vi "Update Overlay.vi"(0 "CaliperType_w_Pic":T9 items=["Distance", "Mid Point", "Perpendicular Projection", "Lines Intersection", "Angle from Horizontal", "Angle from Vertical", "Angle Defined by 3 Points", "Angle Defined by 4 Points", "Bissecting Line", "Mid Line", "Center of Mass", "Area", "Line Fit", "Circle Fit", "Ellipse Fit"], 1 "Vision_Image 2":T2(plugin-control), 5 "Analysis_Point_Result Out":T8[](array[typedef]), 7 "FilteredCaliperEntry":T5[](array[typedef]) {"CaliperType" items=["Distance", "Mid Point", "Perpendicular Projection", "Lines Intersection", "Angle from Horizontal", "Angle from Vertical", "Angle Defined by 3 Points", "Angle Defined by 4 Points", "Bissecting Line", "Mid Line", "Center of Mass", "Area", "Line Fit", "Circle Fit", "Ellipse Fit"]}, 9 "SelectionList 2":T3[](array[typedef]), 12 "Result 2":T1) -> (3 "Image Out":T2)   [LabVIEW 2019]
uses:
  Controls/CaliperType with Picture.ctl
  Analysis/Controls/Analysis_Result_To_Caliper.ctl
  Controls/CaliperDataEntry_SinglePoint.ctl
  Controls/CaliperType.ctl
  Controls/SelectionListEntry.ctl
  Controls/SelectionListEntryPointType.ctl
  Controls/CaliperResult_SinglePoint.ctl
  <vilib>/vision/Image Controls.llb/IMAQ Image.ctl
  Controls/CaliperResult.ctl
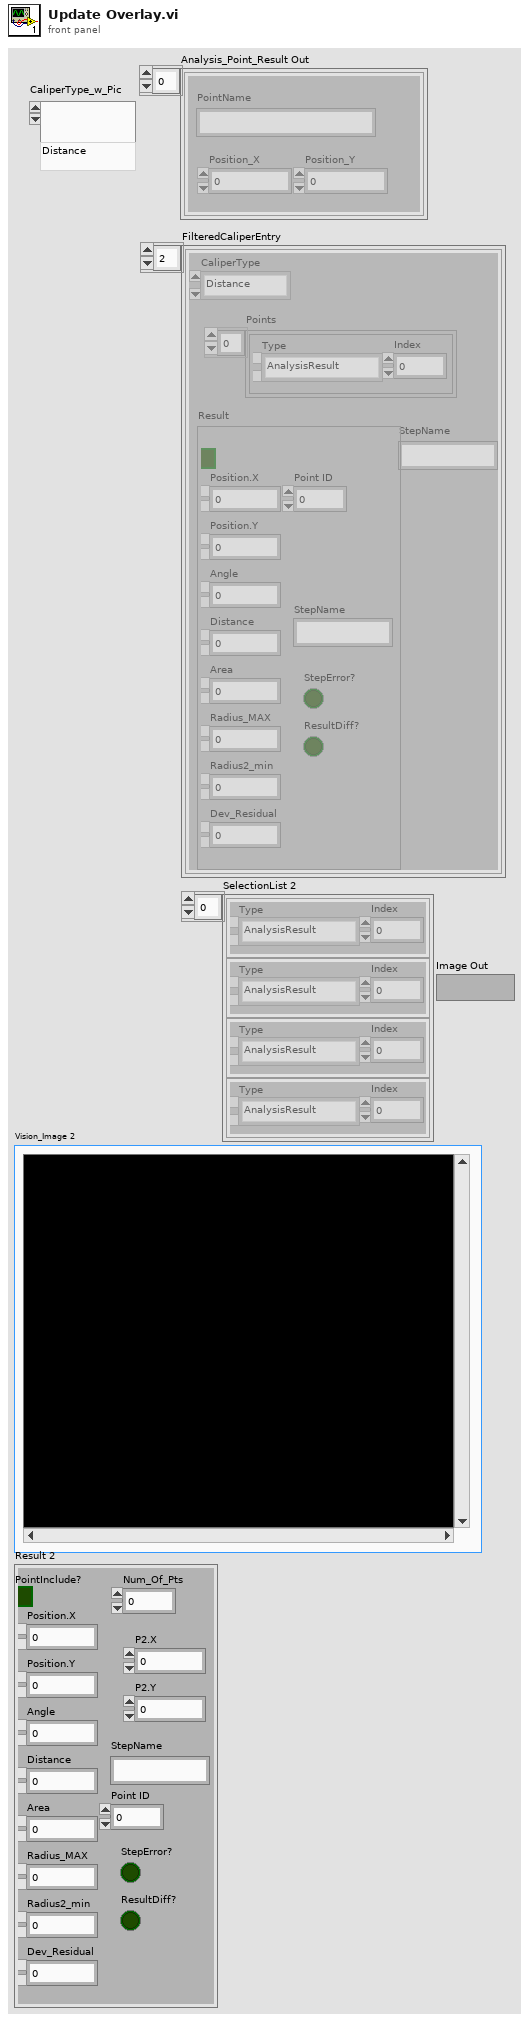
[diagram p1: front panel]
types:
  T1 = typedef "CaliperResult.ctl" = cluster{"PointInclude?":bool, "Num_Of_Pts":u8, "Position.X":dbl, "Position.Y":dbl, "Angle":dbl, "Distance":dbl, "Area":dbl, "Radius_MAX":dbl, "Radius2_min":dbl, "Dev_Residual":dbl, "P2.X":dbl, "P2.Y":dbl, "StepName":string, "Point ID":u8, "StepError?":bool, "ResultDiff?":bool}
  T2 = typedef "IMAQ Image.ctl" = refnum<image>
  T3 = typedef "SelectionListEntry.ctl" = cluster{"Type":T4, "Index":i32}
  T4 = typedef "SelectionListEntryPointType.ctl" = enum16{"AnalysisResult", "CaliperResult"}
  T5 = typedef "CaliperDataEntry_SinglePoint.ctl" = cluster{"CaliperType":T6, "Points":T3[], "Result":T7, "StepName":string}
  T6 = typedef "CaliperType.ctl" = u32
  T7 = typedef "CaliperResult_SinglePoint.ctl" = cluster{"PointInclude?":bool, "Position.X":dbl, "Position.Y":dbl, "Angle":dbl, "Distance":dbl, "Area":dbl, "Radius_MAX":dbl, "Radius2_min":dbl, "Dev_Residual":dbl, "StepName":string, "Point ID":u8, "StepError?":bool, "ResultDiff?":bool}
  T8 = typedef "Analysis_Result_To_Caliper.ctl" = cluster{"PointName":string, "Position_X":dbl, "Position_Y":dbl}
  T9 = typedef "CaliperType with Picture.ctl" = u32
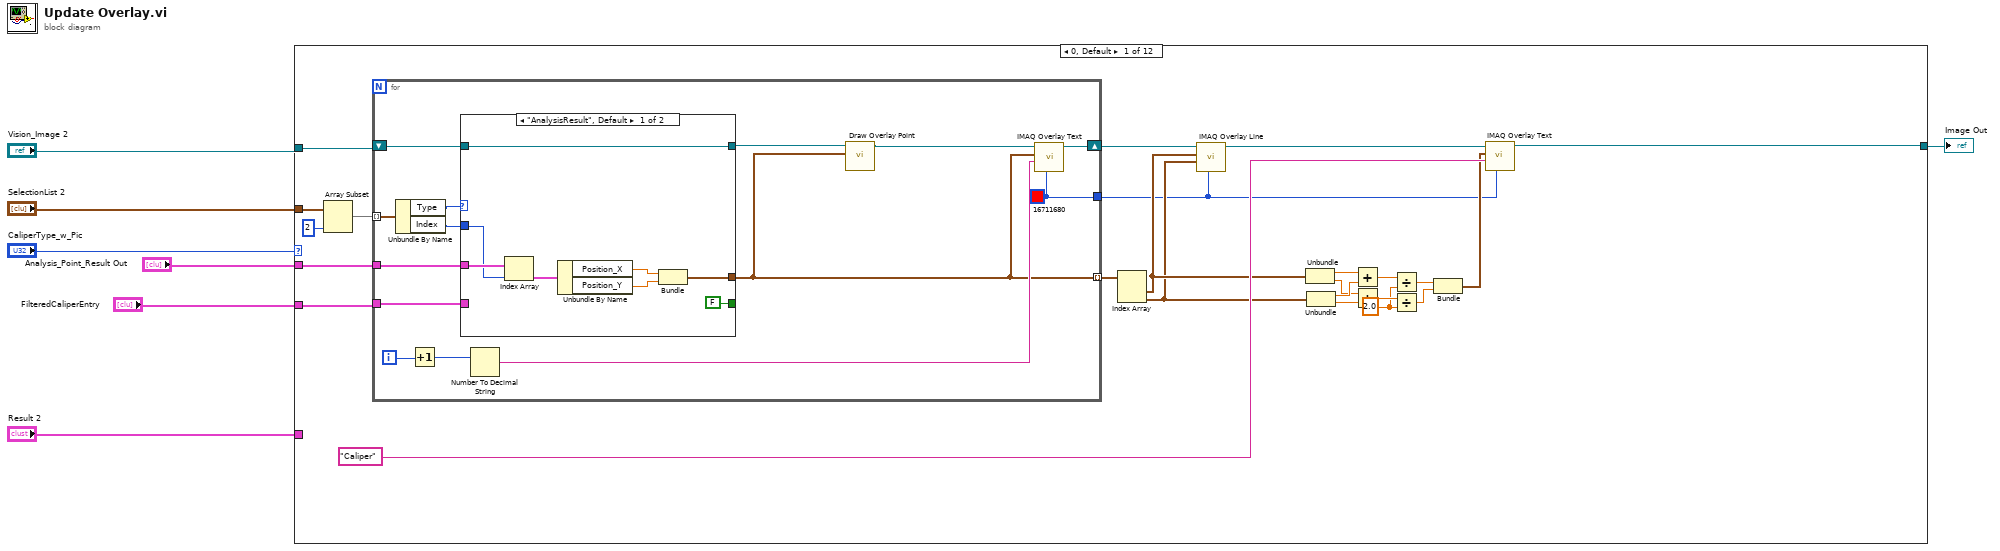
[diagram p0: block diagram]
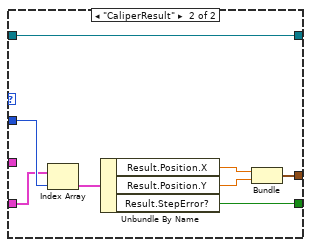
[diagram p2: hidden frame]
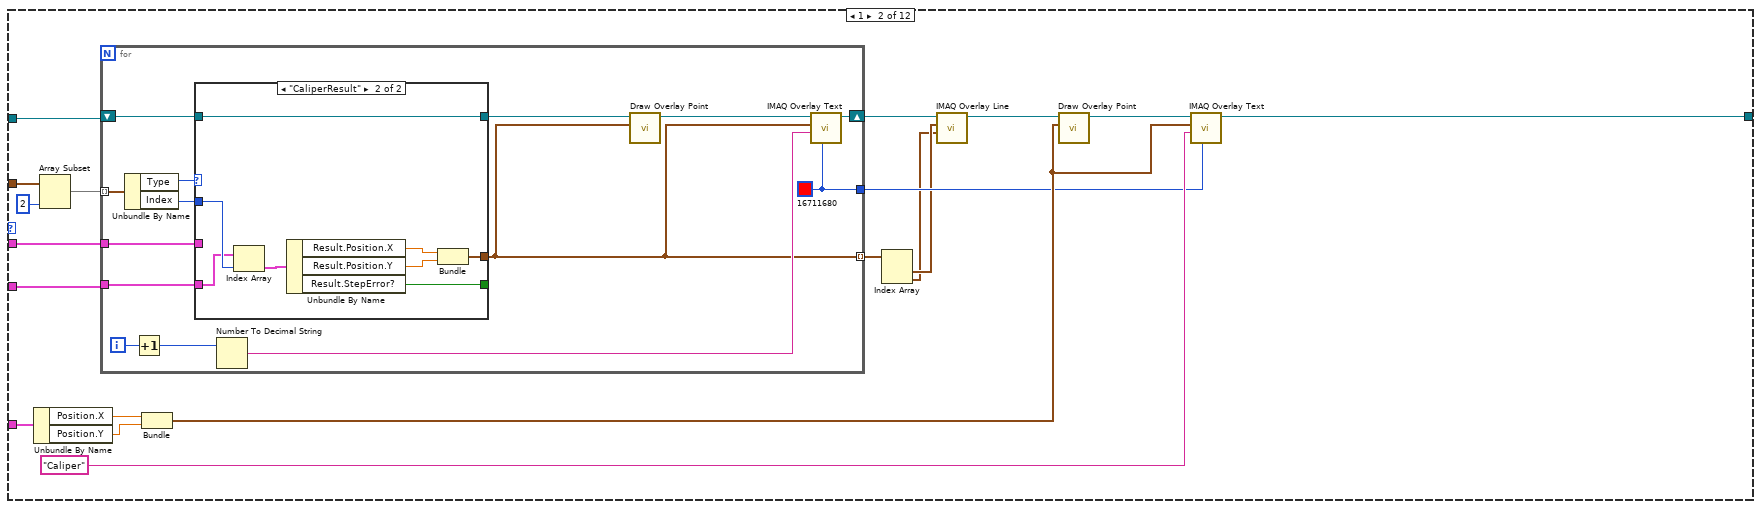
[diagram p3: hidden frame]
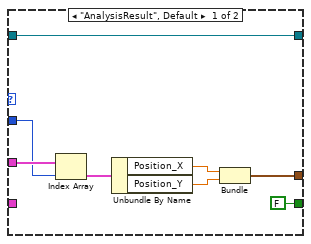
[diagram p4: hidden frame]
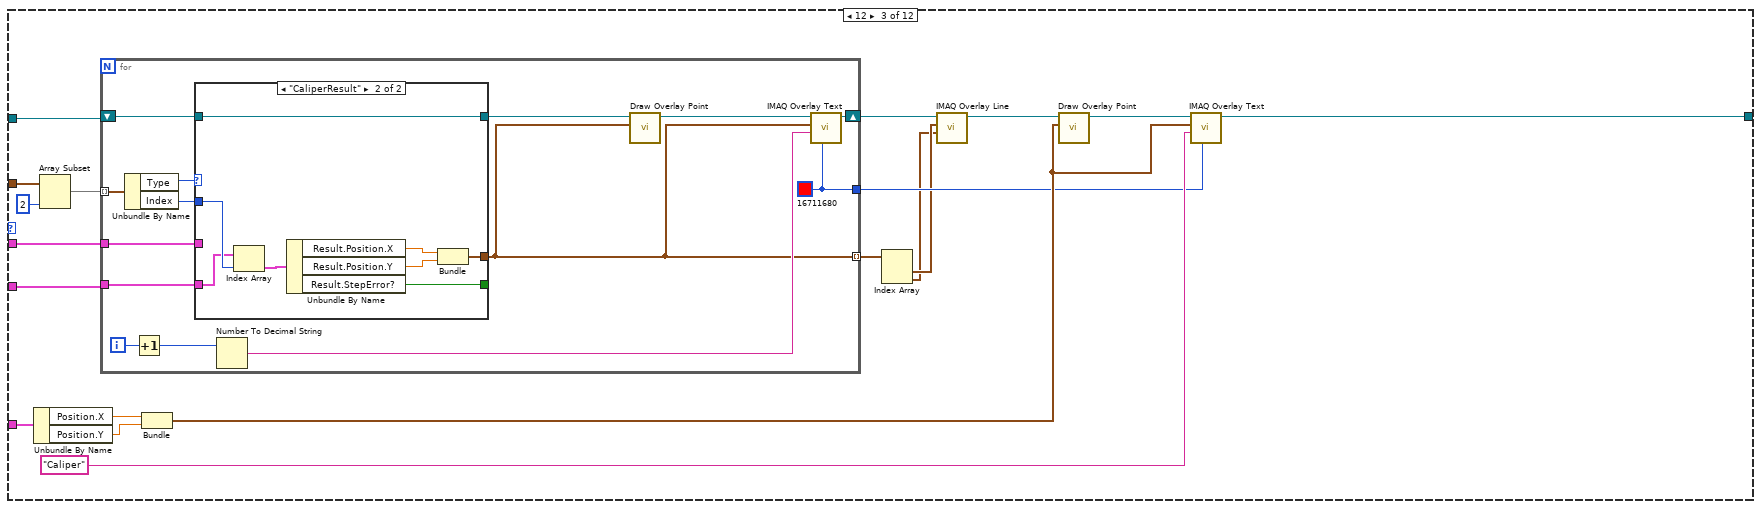
[diagram p5: hidden frame]
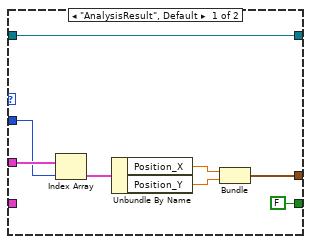
[diagram p6: hidden frame]
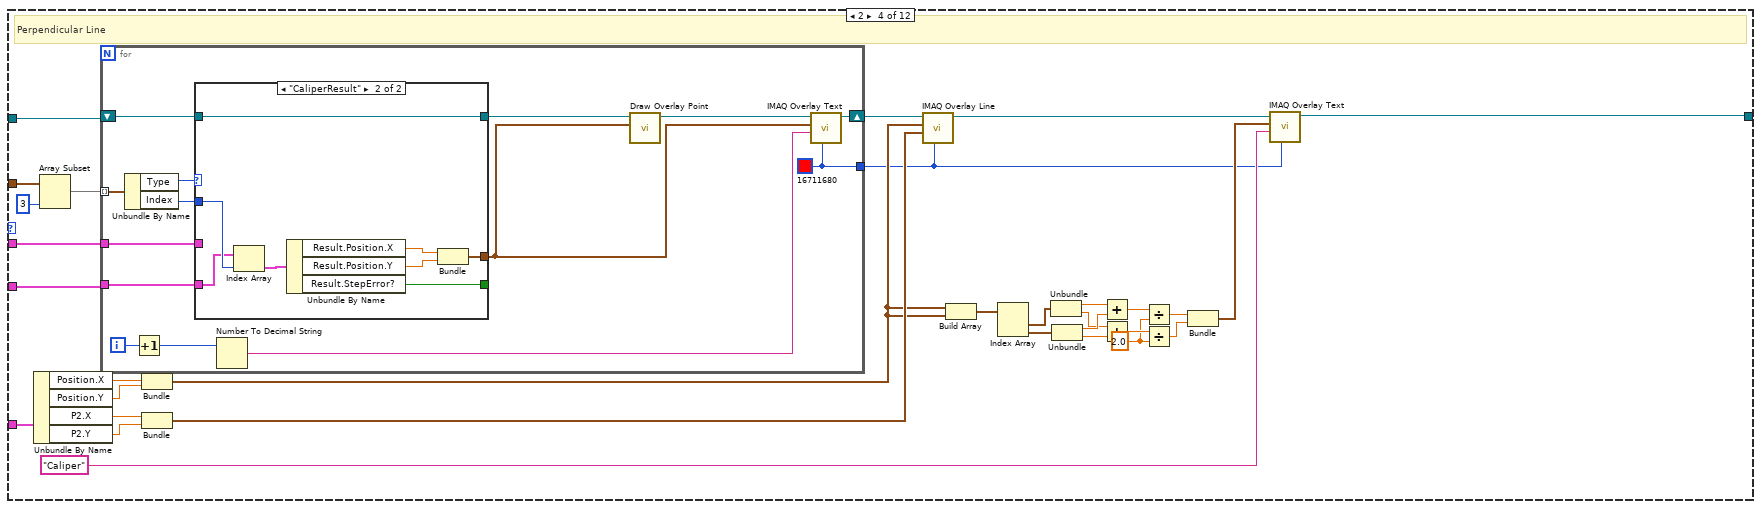
[diagram p7: hidden frame]
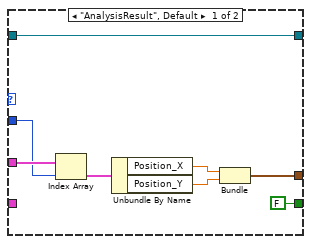
[diagram p8: hidden frame]
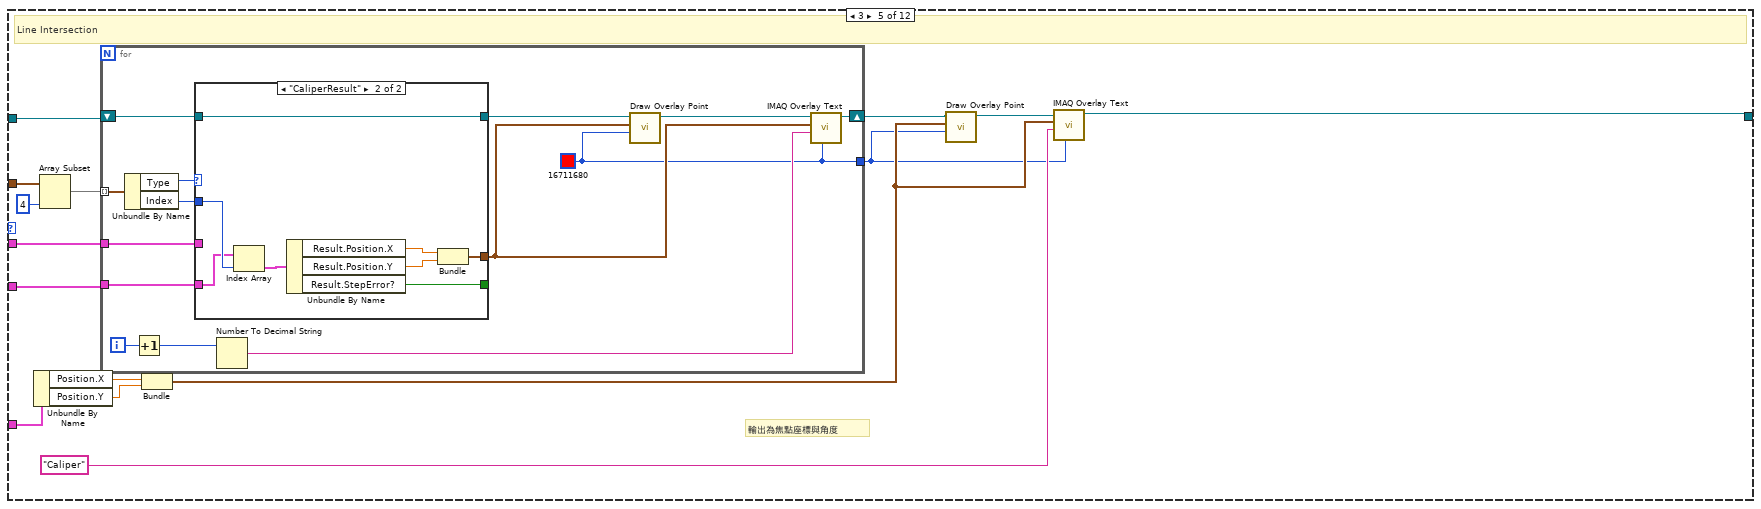
[diagram p9: hidden frame]
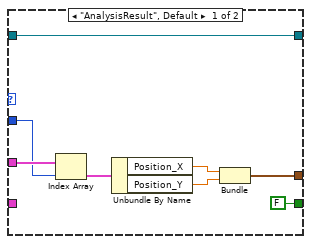
[diagram p10: hidden frame]
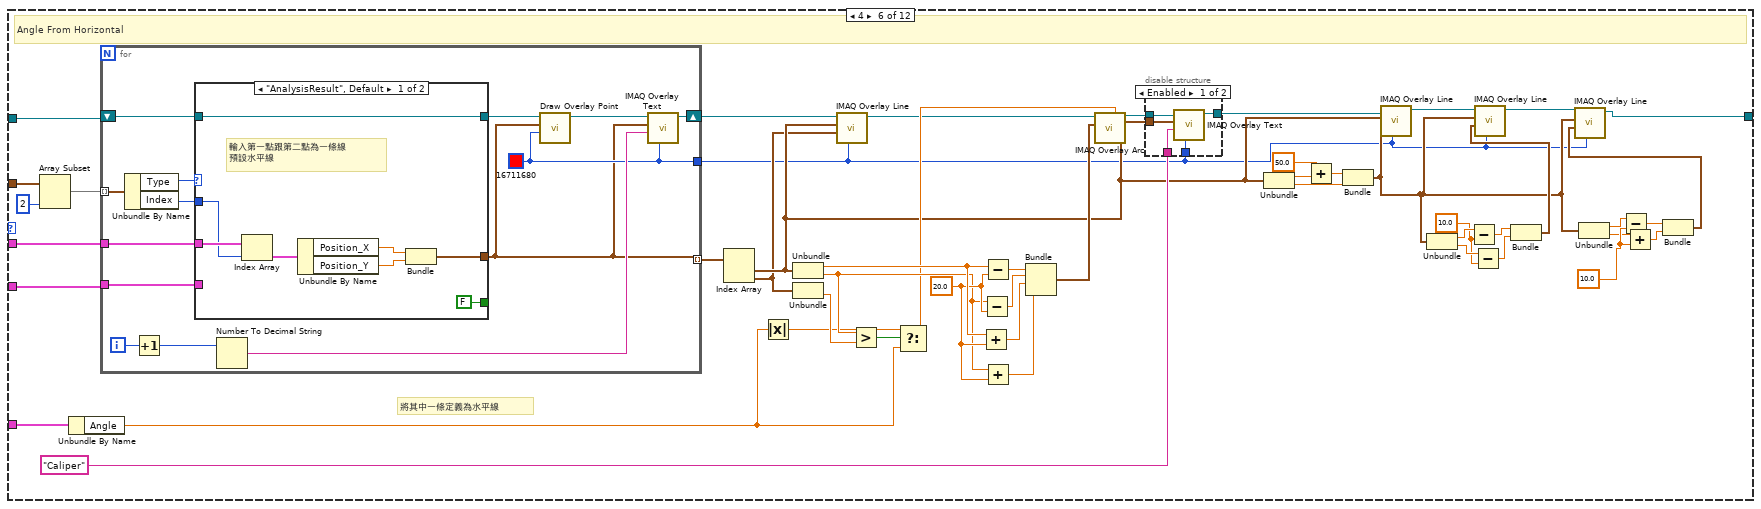
[diagram p11: hidden frame]
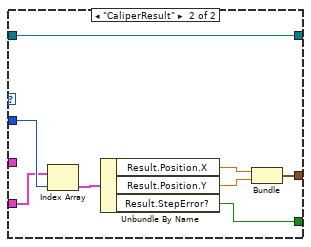
[diagram p13: hidden frame]
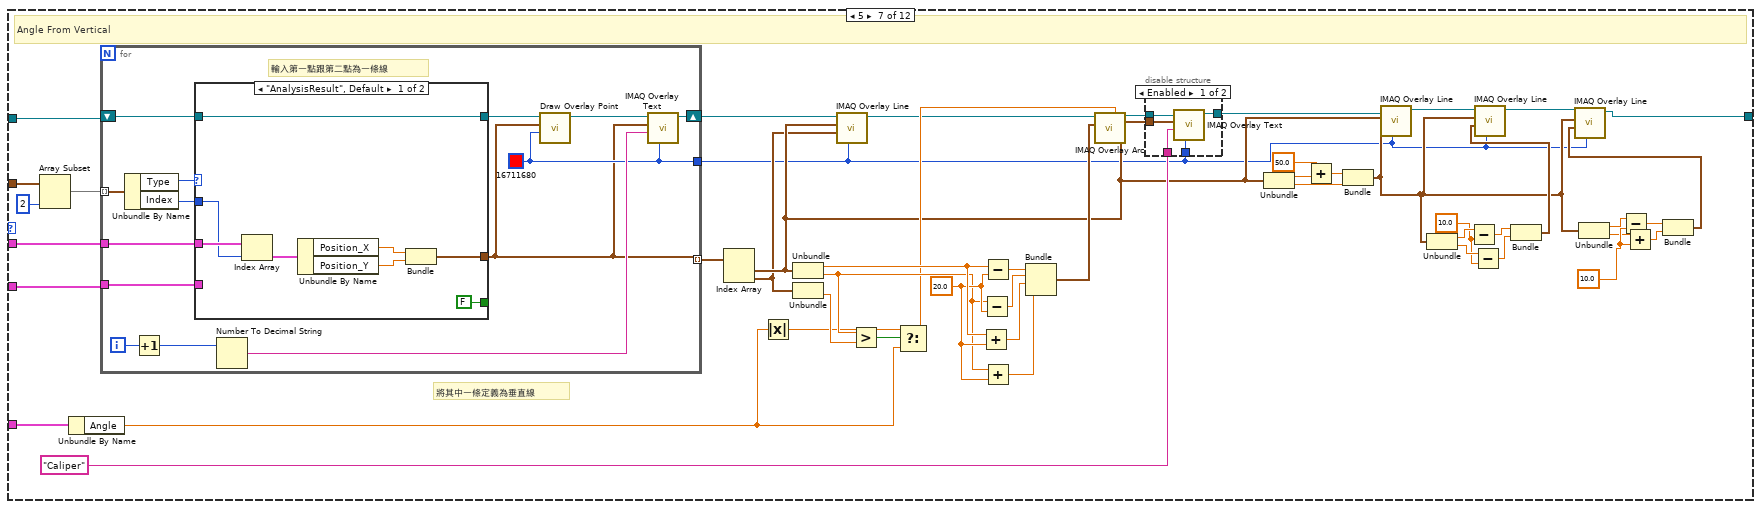
[diagram p14: hidden frame]
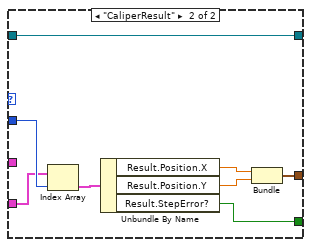
[diagram p16: hidden frame]
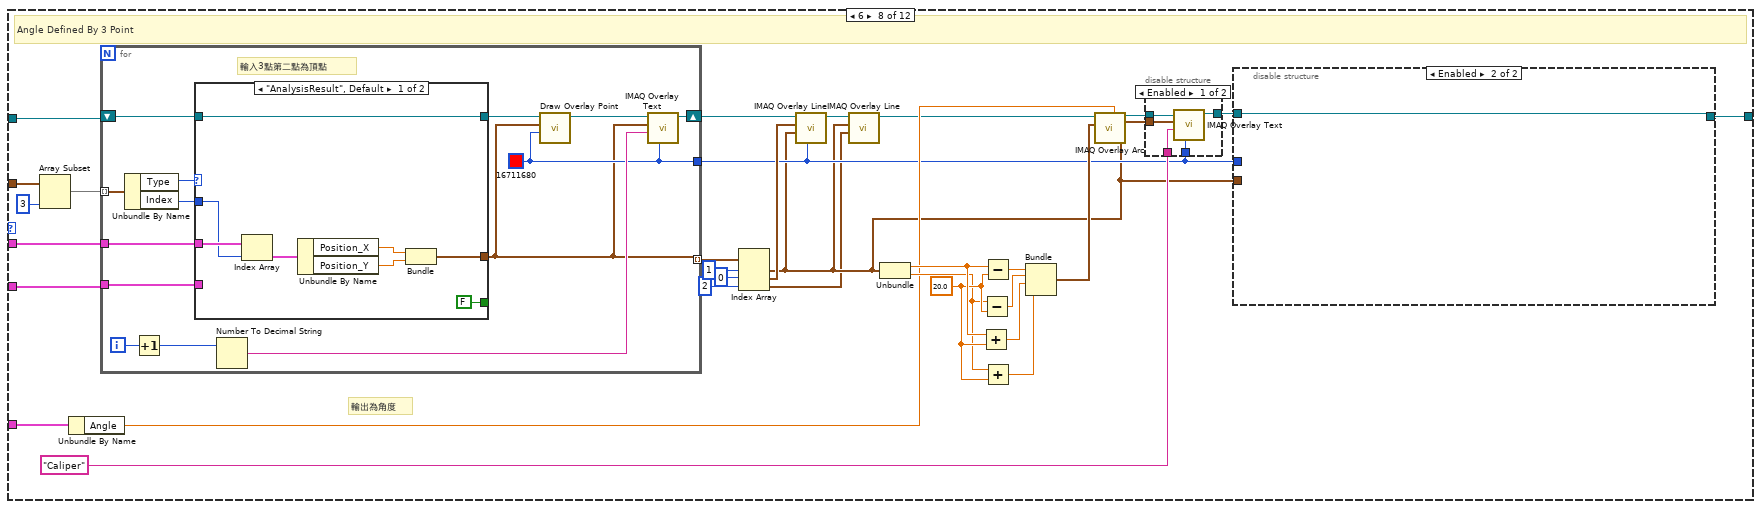
[diagram p17: hidden frame]
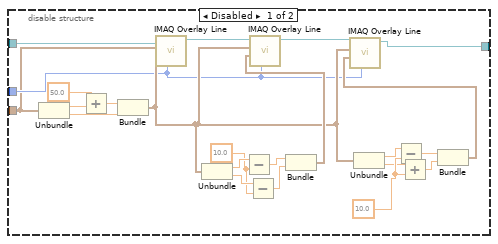
[diagram p18: hidden frame]
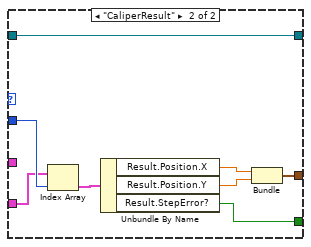
[diagram p20: hidden frame]
diagram:
  n1 = case shown="0, Default" "CaliperType_w_Pic" {
    tunnel: "SelectionList 2" -> [w29 w78 w127 w188 w233 w312 w397 w464 w542 w609 w676 w740]
    tunnel: "Analysis_Point_Result Out" -> [w28 w77 w126 w187 w232 w311 w396 w463 w541 w608 w675 w739]
    tunnel: "FilteredCaliperEntry" -> [w27 w76 w125 w186 w231 w310 w395 w462 w540 w607 w674 w738]
    tunnel: "Vision_Image 2" -> [w26 w67 w116 w182 w229 w308 w393 w460 w538 w605 w672 w736]
    tunnel: [w24 w70 w119 w176 w224 w289 w374 w448 w528 w593 w660 w726] -> w3
    tunnel: "Result 2" -> [_ w75 w124 w185 w230 w309 w394 w461 w539 w606 w673 w737]
    frame 0, Default {
      w15 = 2.0 ("y")
      n2 = Array Subset(array=w29, length=2) -> (w30:T3[])  [unwired: 1 in]
      n3 = for {
        tunnel: w30 -> [w45] mode=indexing
        tunnel: w28 -> [w43]
        tunnel: w27 -> [w41]
        shift-right: [w39] -> w25
        shift-left: w26 -> [w40]
        tunnel: [w33] -> w16 mode=indexing
        tunnel: [w32] -> w8
        i -> [w38]
        w32 = u32 16711680 ("Text Color (black)")
        n4 = Unbundle By Name(w45) -> ("Type"=w44:T4, "Index"=w42:i32)
        n5 = Increment(x=w38) -> (x+1=w37:i32)
        n6 = case shown="\"AnalysisResult\", Default" w44 {
          tunnel: w43 -> [w53 _]
          tunnel: w42 -> [w52 w61]
          tunnel: [w48 w57] -> w33
          tunnel: w41 -> [_ w56]
          tunnel: [FALSE ("StepError?") w55] -> _
          tunnel: w40 -> [w46 w54]
          tunnel: [w46 w54] -> w35
          frame "AnalysisResult", Default {
            n7 = Index Array(array=w53, index=w52) -> (element=w51:T8)
            n8 = Unbundle By Name(w51) -> ("Position_X"=w50:dbl, "Position_Y"=w49:dbl)
            n9 = Bundle("Position_X"=w50, "Position_Y"=w49) -> (w48:cluster{"Position_X":dbl, "Position_Y":dbl})  [unwired: 1 in]
          }
          frame "CaliperResult" {
            n10 = Index Array(array=w56, index=w61) -> (element=w60:T5)
            n11 = Unbundle By Name(w60) -> ("Result.Position.X"=w59:dbl, "Result.Position.Y"=w58:dbl, "Result.StepError?"=w55:bool)
            n12 = Bundle("Position.X"=w59, "Position.Y"=w58) -> (w57:cluster{"Position.X":dbl, "Position.Y":dbl})  [unwired: 1 in]
          }
        }
        n13 = Number To Decimal String(number=w37) -> (decimal integer string=w36:string)  [unwired: 1 in]
        n14 = call "Draw Overlay Point.vi"("Cluster"=w33, "Refnum in"=w35) -> ("Refnum out"=w34:T2)  [unwired: 9 in]
        n15 = call "IMAQ Overlay Text"("Text Color (black)"=w32, "String"=w36, "Origin"=w33, "Image"=w34) -> ("Image Out"=w39:T2)  [unwired: 6 in, 1 out]
      }
      n16 = Index Array(array=w16) -> (element #1=w10:cluster{"Position.X":dbl, "Position.Y":dbl}, element #2=w9:cluster{"Position.X":dbl, "Position.Y":dbl})  [unwired: 2 in]
      n17 = call "IMAQ Overlay Line"("Color"=w8, "End Point"=w9, "Start Point"=w10, "Image"=w25) -> ("Image Out"=w11:T2)  [unwired: 6 in, 1 out]
      n18 = Unbundle(w10) -> ("Position.X"=w22:dbl, "Position.Y"=w19:dbl)
      n19 = Unbundle(w9) -> ("Position.X"=w20:dbl, "Position.Y"=w21:dbl)
      n20 = Add(x=w22, y=w20) -> (x+y=w18:dbl)
      n21 = Add(x=w19, y=w21) -> (x+y=w17:dbl)
      n22 = Divide(x=w18, y=w15) -> (x/y=w14:dbl)
      n23 = Divide(x=w17, y=w15) -> (x/y=w13:dbl)
      n24 = Bundle(w14, w13) -> (w12:cluster{dbl, dbl})  [unwired: 1 in]
      n25 = call "IMAQ Overlay Text"("Text Color (black)"=w8, "String"="Caliper", "Origin"=w12, "Image"=w11) -> ("Image Out"=w24:T2)  [unwired: 6 in, 1 out]
    }
    frame 1 {
      n26 = Unbundle By Name(w75) -> ("Position.X"=w74:dbl, "Position.Y"=w73:dbl)
      n27 = Array Subset(array=w78, length=2) -> (w79:T3[])  [unwired: 1 in]
      n28 = for {
        tunnel: w79 -> [w94] mode=indexing
        tunnel: w77 -> [w92]
        tunnel: w76 -> [w90]
        shift-right: [w86] -> w72
        shift-left: w67 -> [w89]
        tunnel: [w82] -> w66
        tunnel: [w81] -> w64 mode=indexing
        i -> [w85]
        w82 = u32 16711680 ("Text Color (black)")
        n29 = Unbundle By Name(w94) -> ("Type"=w93:T4, "Index"=w91:i32)
        n30 = Increment(x=w85) -> (x+1=w83:i32)
        n31 = case shown="\"CaliperResult\"" w93 {
          tunnel: w92 -> [w102 _]
          tunnel: w91 -> [w101 w110]
          tunnel: [w97 w106] -> w81
          tunnel: w90 -> [_ w105]
          tunnel: [FALSE ("StepError?") w104] -> _
          tunnel: w89 -> [w95 w103]
          tunnel: [w95 w103] -> w88
          frame "AnalysisResult", Default {
            n32 = Index Array(array=w102, index=w101) -> (element=w100:T8)
            n33 = Unbundle By Name(w100) -> ("Position_X"=w99:dbl, "Position_Y"=w98:dbl)
            n34 = Bundle("Position_X"=w99, "Position_Y"=w98) -> (w97:cluster{"Position_X":dbl, "Position_Y":dbl})  [unwired: 1 in]
          }
          frame "CaliperResult" {
            n35 = Index Array(array=w105, index=w110) -> (element=w109:T5)
            n36 = Unbundle By Name(w109) -> ("Result.Position.X"=w108:dbl, "Result.Position.Y"=w107:dbl, "Result.StepError?"=w104:bool)
            n37 = Bundle("Position.X"=w108, "Position.Y"=w107) -> (w106:cluster{"Position.X":dbl, "Position.Y":dbl})  [unwired: 1 in]
          }
        }
        n38 = Number To Decimal String(number=w83) -> (decimal integer string=w84:string)  [unwired: 1 in]
        n39 = call "Draw Overlay Point.vi"("Cluster"=w81, "Refnum in"=w88) -> ("Refnum out"=w87:T2)  [unwired: 9 in]
        n40 = call "IMAQ Overlay Text"("Text Color (black)"=w82, "String"=w84, "Origin"=w81, "Image"=w87) -> ("Image Out"=w86:T2)  [unwired: 6 in, 1 out]
      }
      n41 = Bundle("Position.X"=w74, "Position.Y"=w73) -> (w69:cluster{"Position.X":dbl, "Position.Y":dbl})  [unwired: 1 in]
      n42 = Index Array(array=w64) -> (element #1=w63:cluster{"Position.X":dbl, "Position.Y":dbl}, element #2=w62:cluster{"Position.X":dbl, "Position.Y":dbl})  [unwired: 2 in]
      n43 = call "IMAQ Overlay Line"("End Point"=w62, "Start Point"=w63, "Image"=w72) -> ("Image Out"=w65:T2)  [unwired: 7 in, 1 out]
      n44 = call "Draw Overlay Point.vi"("Cluster"=w69, "Refnum in"=w65) -> ("Refnum out"=w71:T2)  [unwired: 9 in]
      n45 = call "IMAQ Overlay Text"("Text Color (black)"=w66, "String"="Caliper", "Origin"=w69, "Image"=w71) -> ("Image Out"=w70:T2)  [unwired: 6 in, 1 out]
    }
    frame 12 {
      n46 = Unbundle By Name(w124) -> ("Position.X"=w123:dbl, "Position.Y"=w122:dbl)
      n47 = Array Subset(array=w127, length=2) -> (w128:T3[])  [unwired: 1 in]
      n48 = for {
        tunnel: w128 -> [w143] mode=indexing
        tunnel: w126 -> [w141]
        tunnel: w125 -> [w139]
        shift-right: [w135] -> w121
        shift-left: w116 -> [w138]
        tunnel: [w131] -> w115
        tunnel: [w130] -> w113 mode=indexing
        i -> [w134]
        w131 = u32 16711680 ("Text Color (black)")
        n49 = Unbundle By Name(w143) -> ("Type"=w142:T4, "Index"=w140:i32)
        n50 = Increment(x=w134) -> (x+1=w132:i32)
        n51 = case shown="\"CaliperResult\"" w142 {
          tunnel: w141 -> [w151 _]
          tunnel: w140 -> [w150 w159]
          tunnel: [w146 w155] -> w130
          tunnel: w139 -> [_ w154]
          tunnel: [FALSE ("StepError?") w153] -> _
          tunnel: w138 -> [w144 w152]
          tunnel: [w144 w152] -> w137
          frame "AnalysisResult", Default {
            n52 = Index Array(array=w151, index=w150) -> (element=w149:T8)
            n53 = Unbundle By Name(w149) -> ("Position_X"=w148:dbl, "Position_Y"=w147:dbl)
            n54 = Bundle("Position_X"=w148, "Position_Y"=w147) -> (w146:cluster{"Position_X":dbl, "Position_Y":dbl})  [unwired: 1 in]
          }
          frame "CaliperResult" {
            n55 = Index Array(array=w154, index=w159) -> (element=w158:T5)
            n56 = Unbundle By Name(w158) -> ("Result.Position.X"=w157:dbl, "Result.Position.Y"=w156:dbl, "Result.StepError?"=w153:bool)
            n57 = Bundle("Position.X"=w157, "Position.Y"=w156) -> (w155:cluster{"Position.X":dbl, "Position.Y":dbl})  [unwired: 1 in]
          }
        }
        n58 = Number To Decimal String(number=w132) -> (decimal integer string=w133:string)  [unwired: 1 in]
        n59 = call "Draw Overlay Point.vi"("Cluster"=w130, "Refnum in"=w137) -> ("Refnum out"=w136:T2)  [unwired: 9 in]
        n60 = call "IMAQ Overlay Text"("Text Color (black)"=w131, "String"=w133, "Origin"=w130, "Image"=w136) -> ("Image Out"=w135:T2)  [unwired: 6 in, 1 out]
      }
      n61 = Bundle("Position.X"=w123, "Position.Y"=w122) -> (w118:cluster{"Position.X":dbl, "Position.Y":dbl})  [unwired: 1 in]
      n62 = Index Array(array=w113) -> (element #1=w112:cluster{"Position.X":dbl, "Position.Y":dbl}, element #2=w111:cluster{"Position.X":dbl, "Position.Y":dbl})  [unwired: 2 in]
      n63 = call "IMAQ Overlay Line"("End Point"=w111, "Start Point"=w112, "Image"=w121) -> ("Image Out"=w114:T2)  [unwired: 7 in, 1 out]
      n64 = call "Draw Overlay Point.vi"("Cluster"=w118, "Refnum in"=w114) -> ("Refnum out"=w120:T2)  [unwired: 9 in]
      n65 = call "IMAQ Overlay Text"("Text Color (black)"=w115, "String"="Caliper", "Origin"=w118, "Image"=w120) -> ("Image Out"=w119:T2)  [unwired: 6 in, 1 out]
    }
    frame 2 {
      w166 = 2.0 ("y")
      # "Perpendicular Line"
      n66 = Unbundle By Name(w185) -> ("Position.X"=w181:dbl, "Position.Y"=w180:dbl, "P2.X"=w184:dbl, "P2.Y"=w183:dbl)
      n67 = Array Subset(array=w188, length=3) -> (w189:T3[])  [unwired: 1 in]
      n68 = for {
        tunnel: w189 -> [w204] mode=indexing
        tunnel: w187 -> [w202]
        tunnel: w186 -> [w200]
        shift-right: [w196] -> w179
        shift-left: w182 -> [w199]
        tunnel: [w191] -> w160
        i -> [w194]
        w191 = u32 16711680 ("Text Color (black)")
        n69 = Unbundle By Name(w204) -> ("Type"=w203:T4, "Index"=w201:i32)
        n70 = Increment(x=w194) -> (x+1=w192:i32)
        n71 = case shown="\"CaliperResult\"" w203 {
          tunnel: w202 -> [w212 _]
          tunnel: w201 -> [w211 w220]
          tunnel: [w207 w216] -> w195
          tunnel: w200 -> [_ w215]
          tunnel: [FALSE ("StepError?") w214] -> _
          tunnel: w199 -> [w205 w213]
          tunnel: [w205 w213] -> w198
          frame "AnalysisResult", Default {
            n72 = Index Array(array=w212, index=w211) -> (element=w210:T8)
            n73 = Unbundle By Name(w210) -> ("Position_X"=w209:dbl, "Position_Y"=w208:dbl)
            n74 = Bundle("Position_X"=w209, "Position_Y"=w208) -> (w207:cluster{"Position_X":dbl, "Position_Y":dbl})  [unwired: 1 in]
          }
          frame "CaliperResult" {
            n75 = Index Array(array=w215, index=w220) -> (element=w219:T5)
            n76 = Unbundle By Name(w219) -> ("Result.Position.X"=w218:dbl, "Result.Position.Y"=w217:dbl, "Result.StepError?"=w214:bool)
            n77 = Bundle("Position.X"=w218, "Position.Y"=w217) -> (w216:cluster{"Position.X":dbl, "Position.Y":dbl})  [unwired: 1 in]
          }
        }
        n78 = Number To Decimal String(number=w192) -> (decimal integer string=w193:string)  [unwired: 1 in]
        n79 = call "Draw Overlay Point.vi"("Cluster"=w195, "Refnum in"=w198) -> ("Refnum out"=w197:T2)  [unwired: 9 in]
        n80 = call "IMAQ Overlay Text"("Text Color (black)"=w191, "String"=w193, "Origin"=w195, "Image"=w197) -> ("Image Out"=w196:T2)  [unwired: 6 in, 1 out]
      }
      n81 = Bundle("Position.X"=w181, "Position.Y"=w180) -> (w175:cluster{"Position.X":dbl, "Position.Y":dbl})  [unwired: 1 in]
      n82 = Bundle("P2.X"=w184, "P2.Y"=w183) -> (w178:cluster{"P2.X":dbl, "P2.Y":dbl})  [unwired: 1 in]
      n83 = call "IMAQ Overlay Line"("Color"=w160, "End Point"=w178, "Start Point"=w175, "Image"=w179) -> ("Image Out"=w177:T2)  [unwired: 6 in, 1 out]
      n84 = Build Array(w175, w175) -> (w163:cluster{"Position.X":dbl, "Position.Y":dbl}[])
      n85 = Index Array(array=w163) -> (element #1=w174:cluster{"Position.X":dbl, "Position.Y":dbl}, element #2=w167:cluster{"Position.X":dbl, "Position.Y":dbl})  [unwired: 2 in]
      n86 = Unbundle(w174) -> ("Position.X"=w173:dbl, "Position.Y"=w170:dbl)
      n87 = Unbundle(w167) -> ("Position.X"=w171:dbl, "Position.Y"=w172:dbl)
      n88 = Add(x=w173, y=w171) -> (x+y=w169:dbl)
      n89 = Add(x=w170, y=w172) -> (x+y=w168:dbl)
      n90 = Divide(x=w169, y=w166) -> (x/y=w165:dbl)
      n91 = Divide(x=w168, y=w166) -> (x/y=w164:dbl)
      n92 = Bundle(w165, w164) -> (w162:cluster{dbl, dbl})  [unwired: 1 in]
      n93 = call "IMAQ Overlay Text"("Text Color (black)"=w160, "String"="Caliper", "Origin"=w162, "Image"=w177) -> ("Image Out"=w176:T2)  [unwired: 6 in, 1 out]
    }
    frame 3 {
      # "輸出為焦點座標與角度"
      # "Line Intersection"
      n94 = Unbundle By Name(w230) -> ("Position.X"=w228:dbl, "Position.Y"=w227:dbl)
      n95 = Array Subset(array=w233, length=4) -> (w234:T3[])  [unwired: 1 in]
      n96 = for {
        tunnel: w234 -> [w249] mode=indexing
        tunnel: w232 -> [w247]
        tunnel: w231 -> [w245]
        shift-right: [w241] -> w226
        shift-left: w229 -> [w244]
        tunnel: [w236] -> w221
        i -> [w239]
        w236 = u32 16711680 ("Text Color (black)")
        n97 = Unbundle By Name(w249) -> ("Type"=w248:T4, "Index"=w246:i32)
        n98 = Increment(x=w239) -> (x+1=w237:i32)
        n99 = case shown="\"CaliperResult\"" w248 {
          tunnel: w247 -> [w257 _]
          tunnel: w246 -> [w256 w265]
          tunnel: [w252 w261] -> w240
          tunnel: w245 -> [_ w260]
          tunnel: [FALSE ("StepError?") w259] -> _
          tunnel: w244 -> [w250 w258]
          tunnel: [w250 w258] -> w243
          frame "AnalysisResult", Default {
            n100 = Index Array(array=w257, index=w256) -> (element=w255:T8)
            n101 = Unbundle By Name(w255) -> ("Position_X"=w254:dbl, "Position_Y"=w253:dbl)
            n102 = Bundle("Position_X"=w254, "Position_Y"=w253) -> (w252:cluster{"Position_X":dbl, "Position_Y":dbl})  [unwired: 1 in]
          }
          frame "CaliperResult" {
            n103 = Index Array(array=w260, index=w265) -> (element=w264:T5)
            n104 = Unbundle By Name(w264) -> ("Result.Position.X"=w263:dbl, "Result.Position.Y"=w262:dbl, "Result.StepError?"=w259:bool)
            n105 = Bundle("Position.X"=w263, "Position.Y"=w262) -> (w261:cluster{"Position.X":dbl, "Position.Y":dbl})  [unwired: 1 in]
          }
        }
        n106 = Number To Decimal String(number=w237) -> (decimal integer string=w238:string)  [unwired: 1 in]
        n107 = call "Draw Overlay Point.vi"("Color"=w236, "Cluster"=w240, "Refnum in"=w243) -> ("Refnum out"=w242:T2)  [unwired: 8 in]
        n108 = call "IMAQ Overlay Text"("Text Color (black)"=w236, "String"=w238, "Origin"=w240, "Image"=w242) -> ("Image Out"=w241:T2)  [unwired: 6 in, 1 out]
      }
      n109 = Bundle("Position.X"=w228, "Position.Y"=w227) -> (w223:cluster{"Position.X":dbl, "Position.Y":dbl})  [unwired: 1 in]
      n110 = call "Draw Overlay Point.vi"("Color"=w221, "Cluster"=w223, "Refnum in"=w226) -> ("Refnum out"=w225:T2)  [unwired: 8 in]
      n111 = call "IMAQ Overlay Text"("Text Color (black)"=w221, "String"="Caliper", "Origin"=w223, "Image"=w225) -> ("Image Out"=w224:T2)  [unwired: 6 in, 1 out]
    }
    frame 4 {
      w277 = 10.0 ("x")
      w279 = 10.0 ("x")
      w302 = 20.0
      # "將其中一條定義為水平線"
      # "Angle From Horizontal"
      n112 = Array Subset(array=w312, length=2) -> (w313:T3[])  [unwired: 1 in]
      n113 = Unbundle By Name(w309) -> ("Angle"=w271:dbl)
      n114 = for {
        tunnel: w313 -> [w334] mode=indexing
        tunnel: w311 -> [w332]
        tunnel: w310 -> [w330]
        shift-right: [w326] -> w306
        shift-left: w308 -> [w329]
        tunnel: [w322] -> w266
        tunnel: [w321] -> w304 mode=indexing
        i -> [w325]
        w322 = u32 16711680 ("Text Color (black)")
        n115 = Unbundle By Name(w334) -> ("Type"=w333:T4, "Index"=w331:i32)
        n116 = Increment(x=w325) -> (x+1=w323:i32)
        n117 = case shown="\"AnalysisResult\", Default" w333 {
          tunnel: w332 -> [w342 _]
          tunnel: w331 -> [w341 w350]
          tunnel: [w337 w346] -> w321
          tunnel: w330 -> [_ w345]
          tunnel: [FALSE ("StepError?") w344] -> _
          tunnel: w329 -> [w335 w343]
          tunnel: [w335 w343] -> w328
          frame "AnalysisResult", Default {
            # "輸入第一點跟第二點為一條線\n預設水平線"
            n118 = Index Array(array=w342, index=w341) -> (element=w340:T8)
            n119 = Unbundle By Name(w340) -> ("Position_X"=w339:dbl, "Position_Y"=w338:dbl)
            n120 = Bundle("Position_X"=w339, "Position_Y"=w338) -> (w337:cluster{"Position_X":dbl, "Position_Y":dbl})  [unwired: 1 in]
          }
          frame "CaliperResult" {
            n121 = Index Array(array=w345, index=w350) -> (element=w349:T5)
            n122 = Unbundle By Name(w349) -> ("Result.Position.X"=w348:dbl, "Result.Position.Y"=w347:dbl, "Result.StepError?"=w344:bool)
            n123 = Bundle("Position.X"=w348, "Position.Y"=w347) -> (w346:cluster{"Position.X":dbl, "Position.Y":dbl})  [unwired: 1 in]
          }
        }
        n124 = Number To Decimal String(number=w323) -> (decimal integer string=w324:string)  [unwired: 1 in]
        n125 = call "Draw Overlay Point.vi"("Color"=w322, "Cluster"=w321, "Refnum in"=w328) -> ("Refnum out"=w327:T2)  [unwired: 8 in]
        n126 = call "IMAQ Overlay Text"("Text Color (black)"=w322, "String"=w324, "Origin"=w321, "Image"=w327) -> ("Image Out"=w326:T2)  [unwired: 6 in, 1 out]
      }
      n127 = Index Array(array=w304) -> (element #1=w268:cluster{"Position.X":dbl, "Position.Y":dbl}, element #2=w267:cluster{"Position.X":dbl, "Position.Y":dbl})  [unwired: 2 in]
      n128 = Absolute Value(x=w271) -> (abs(x)=w272:dbl)
      n129 = Unbundle(w268) -> ("Position.X"=w303:dbl, "Position.Y"=w275:dbl)
      n130 = Unbundle(w267) -> ("Position.Y"=w274:dbl)  [unwired: 1 out]
      n131 = call "IMAQ Overlay Line"("Color"=w266, "End Point"=w267, "Start Point"=w268, "Image"=w306) -> ("Image Out"=w269:T2)  [unwired: 6 in, 1 out]
      n132 = Greater?(x=w275, y=w274) -> (0:w273:bool)
      n133 = Select(t=w272, s=w273, f=w271) -> (s? t:f=w270:dbl)
      n134 = Add(x=w303, y=w302) -> (x+y=w299:dbl)
      n135 = Subtract(x=w275, y=w302) -> (x-y=w300:dbl)
      n136 = Subtract(x=w303, y=w302) -> (x-y=w301:dbl)
      n137 = Add(x=w275, y=w302) -> (x+y=w298:dbl)
      n138 = Bundle(w301, w300, w299, w298) -> (w297:cluster{dbl, dbl, dbl, dbl})  [unwired: 1 in]
      n139 = call "IMAQ Overlay Arc"("End Angle (degrees)"=w270, "Bounding Rectangle"=w297, "Image"=w269) -> ("Image Out"=w305:T2)  [unwired: 7 in, 1 out]
      n140 = disable-structure shown="Enabled" {
        disable-tunnel: [w319 w320] -> w296
        disable-tunnel: "Caliper" -> [w318 _]
        disable-tunnel: w266 -> [w317 _]
        disable-tunnel: w305 -> [w316 w320]
        disable-tunnel: w268 -> [w315 _]
        frame Enabled {
          n141 = call "IMAQ Overlay Text"("Text Color (black)"=w317, "String"=w318, "Origin"=w315, "Image"=w316) -> ("Image Out"=w319:T2)  [unwired: 6 in, 1 out]
        }
        frame Disabled {
        }
      }
      n142 = Unbundle(w268) -> ("Position.X"=w295:dbl, "Position.Y"=w292:dbl)
      n143 = Add(x=50.0, y=w295) -> (x+y=w293:dbl)
      n144 = Bundle(w293, "Position.Y"=w292) -> (w282:cluster{dbl, "Position.Y":dbl})  [unwired: 1 in]
      n145 = call "IMAQ Overlay Line"("Color"=w266, "End Point"=w282, "Start Point"=w268, "Image"=w296) -> ("Image Out"=w291:T2)  [unwired: 6 in, 1 out]
      n146 = Unbundle(w282) -> (w281:dbl, "Position.Y"=w280:dbl)
      n147 = Subtract(x=w281, y=w279) -> (x-y=w288:dbl)
      n148 = Subtract(x=w280, y=w279) -> (x-y=w287:dbl)
      n149 = Bundle(w288, w287) -> (w286:cluster{dbl, dbl})  [unwired: 1 in]
      n150 = call "IMAQ Overlay Line"("Color"=w266, "End Point"=w286, "Start Point"=w282, "Image"=w291) -> ("Image Out"=w290:T2)  [unwired: 6 in, 1 out]
      n151 = Unbundle(w282) -> (w278:dbl, "Position.Y"=w276:dbl)
      n152 = Subtract(x=w278, y=w277) -> (x-y=w284:dbl)
      n153 = Add(x=w276, y=w277) -> (x+y=w285:dbl)
      n154 = Bundle(w284, w285) -> (w283:cluster{dbl, dbl})  [unwired: 1 in]
      n155 = call "IMAQ Overlay Line"("Color"=w266, "End Point"=w283, "Start Point"=w282, "Image"=w290) -> ("Image Out"=w289:T2)  [unwired: 6 in, 1 out]
    }
    frame 5 {
      w362 = 10.0 ("x")
      w364 = 10.0 ("x")
      w387 = 20.0
      # "將其中一條定義為垂直線"
      # "Angle From Vertical"
      n156 = Array Subset(array=w397, length=2) -> (w398:T3[])  [unwired: 1 in]
      n157 = Unbundle By Name(w394) -> ("Angle"=w356:dbl)
      n158 = for {
        tunnel: w398 -> [w419] mode=indexing
        tunnel: w396 -> [w417]
        tunnel: w395 -> [w415]
        shift-right: [w411] -> w391
        shift-left: w393 -> [w414]
        tunnel: [w407] -> w351
        tunnel: [w406] -> w389 mode=indexing
        i -> [w410]
        w407 = u32 16711680 ("Text Color (black)")
        # "輸入第一點跟第二點為一條線"
        n159 = Unbundle By Name(w419) -> ("Type"=w418:T4, "Index"=w416:i32)
        n160 = Increment(x=w410) -> (x+1=w408:i32)
        n161 = case shown="\"AnalysisResult\", Default" w418 {
          tunnel: w417 -> [w427 _]
          tunnel: w416 -> [w426 w435]
          tunnel: [w422 w431] -> w406
          tunnel: w415 -> [_ w430]
          tunnel: [FALSE ("StepError?") w429] -> _
          tunnel: w414 -> [w420 w428]
          tunnel: [w420 w428] -> w413
          frame "AnalysisResult", Default {
            n162 = Index Array(array=w427, index=w426) -> (element=w425:T8)
            n163 = Unbundle By Name(w425) -> ("Position_X"=w424:dbl, "Position_Y"=w423:dbl)
            n164 = Bundle("Position_X"=w424, "Position_Y"=w423) -> (w422:cluster{"Position_X":dbl, "Position_Y":dbl})  [unwired: 1 in]
          }
          frame "CaliperResult" {
            n165 = Index Array(array=w430, index=w435) -> (element=w434:T5)
            n166 = Unbundle By Name(w434) -> ("Result.Position.X"=w433:dbl, "Result.Position.Y"=w432:dbl, "Result.StepError?"=w429:bool)
            n167 = Bundle("Position.X"=w433, "Position.Y"=w432) -> (w431:cluster{"Position.X":dbl, "Position.Y":dbl})  [unwired: 1 in]
          }
        }
        n168 = Number To Decimal String(number=w408) -> (decimal integer string=w409:string)  [unwired: 1 in]
        n169 = call "Draw Overlay Point.vi"("Color"=w407, "Cluster"=w406, "Refnum in"=w413) -> ("Refnum out"=w412:T2)  [unwired: 8 in]
        n170 = call "IMAQ Overlay Text"("Text Color (black)"=w407, "String"=w409, "Origin"=w406, "Image"=w412) -> ("Image Out"=w411:T2)  [unwired: 6 in, 1 out]
      }
      n171 = Index Array(array=w389) -> (element #1=w353:cluster{"Position.X":dbl, "Position.Y":dbl}, element #2=w352:cluster{"Position.X":dbl, "Position.Y":dbl})  [unwired: 2 in]
      n172 = Absolute Value(x=w356) -> (abs(x)=w357:dbl)
      n173 = Unbundle(w353) -> ("Position.X"=w388:dbl, "Position.Y"=w360:dbl)
      n174 = Unbundle(w352) -> ("Position.Y"=w359:dbl)  [unwired: 1 out]
      n175 = call "IMAQ Overlay Line"("Color"=w351, "End Point"=w352, "Start Point"=w353, "Image"=w391) -> ("Image Out"=w354:T2)  [unwired: 6 in, 1 out]
      n176 = Greater?(x=w360, y=w359) -> (0:w358:bool)
      n177 = Select(t=w357, s=w358, f=w356) -> (s? t:f=w355:dbl)
      n178 = Add(x=w388, y=w387) -> (x+y=w384:dbl)
      n179 = Subtract(x=w360, y=w387) -> (x-y=w385:dbl)
      n180 = Subtract(x=w388, y=w387) -> (x-y=w386:dbl)
      n181 = Add(x=w360, y=w387) -> (x+y=w383:dbl)
      n182 = Bundle(w386, w385, w384, w383) -> (w382:cluster{dbl, dbl, dbl, dbl})  [unwired: 1 in]
      n183 = call "IMAQ Overlay Arc"("End Angle (degrees)"=w355, "Bounding Rectangle"=w382, "Image"=w354) -> ("Image Out"=w390:T2)  [unwired: 7 in, 1 out]
      n184 = disable-structure shown="Enabled" {
        disable-tunnel: [w404 w405] -> w381
        disable-tunnel: "Caliper" -> [w403 _]
        disable-tunnel: w351 -> [w402 _]
        disable-tunnel: w390 -> [w401 w405]
        disable-tunnel: w353 -> [w400 _]
        frame Enabled {
          n185 = call "IMAQ Overlay Text"("Text Color (black)"=w402, "String"=w403, "Origin"=w400, "Image"=w401) -> ("Image Out"=w404:T2)  [unwired: 6 in, 1 out]
        }
        frame Disabled {
        }
      }
      n186 = Unbundle(w353) -> ("Position.X"=w380:dbl, "Position.Y"=w377:dbl)
      n187 = Add(x=50.0, y=w380) -> (x+y=w378:dbl)
      n188 = Bundle(w378, "Position.Y"=w377) -> (w367:cluster{dbl, "Position.Y":dbl})  [unwired: 1 in]
      n189 = call "IMAQ Overlay Line"("Color"=w351, "End Point"=w367, "Start Point"=w353, "Image"=w381) -> ("Image Out"=w376:T2)  [unwired: 6 in, 1 out]
      n190 = Unbundle(w367) -> (w366:dbl, "Position.Y"=w365:dbl)
      n191 = Subtract(x=w366, y=w364) -> (x-y=w373:dbl)
      n192 = Subtract(x=w365, y=w364) -> (x-y=w372:dbl)
      n193 = Bundle(w373, w372) -> (w371:cluster{dbl, dbl})  [unwired: 1 in]
      n194 = call "IMAQ Overlay Line"("Color"=w351, "End Point"=w371, "Start Point"=w367, "Image"=w376) -> ("Image Out"=w375:T2)  [unwired: 6 in, 1 out]
      n195 = Unbundle(w367) -> (w363:dbl, "Position.Y"=w361:dbl)
      n196 = Subtract(x=w363, y=w362) -> (x-y=w369:dbl)
      n197 = Add(x=w361, y=w362) -> (x+y=w370:dbl)
      n198 = Bundle(w369, w370) -> (w368:cluster{dbl, dbl})  [unwired: 1 in]
      n199 = call "IMAQ Overlay Line"("Color"=w351, "End Point"=w368, "Start Point"=w367, "Image"=w375) -> ("Image Out"=w374:T2)  [unwired: 6 in, 1 out]
    }
    frame 6 {
      w455 = 20.0
      # "輸出為角度"
      # "Angle Defined By 3 Point"
      n200 = Array Subset(array=w464, length=3) -> (w465:T3[])  [unwired: 1 in]
      n201 = Unbundle By Name(w461) -> ("Angle"=w445:dbl)
      n202 = for {
        tunnel: w465 -> [w510] mode=indexing
        tunnel: w463 -> [w508]
        tunnel: w462 -> [w506]
        shift-right: [w502] -> w446
        shift-left: w460 -> [w505]
        tunnel: [w498] -> w439
        tunnel: [w497] -> w457 mode=indexing
        i -> [w501]
        w498 = u32 16711680 ("Text Color (black)")
        # "輸入3點第二點為頂點"
        n203 = Unbundle By Name(w510) -> ("Type"=w509:T4, "Index"=w507:i32)
        n204 = Increment(x=w501) -> (x+1=w499:i32)
        n205 = case shown="\"AnalysisResult\", Default" w509 {
          tunnel: w508 -> [w518 _]
          tunnel: w507 -> [w517 w526]
          tunnel: [w513 w522] -> w497
          tunnel: w506 -> [_ w521]
          tunnel: [FALSE ("StepError?") w520] -> _
          tunnel: w505 -> [w511 w519]
          tunnel: [w511 w519] -> w504
          frame "AnalysisResult", Default {
            n206 = Index Array(array=w518, index=w517) -> (element=w516:T8)
            n207 = Unbundle By Name(w516) -> ("Position_X"=w515:dbl, "Position_Y"=w514:dbl)
            n208 = Bundle("Position_X"=w515, "Position_Y"=w514) -> (w513:cluster{"Position_X":dbl, "Position_Y":dbl})  [unwired: 1 in]
          }
          frame "CaliperResult" {
            n209 = Index Array(array=w521, index=w526) -> (element=w525:T5)
            n210 = Unbundle By Name(w525) -> ("Result.Position.X"=w524:dbl, "Result.Position.Y"=w523:dbl, "Result.StepError?"=w520:bool)
            n211 = Bundle("Position.X"=w524, "Position.Y"=w523) -> (w522:cluster{"Position.X":dbl, "Position.Y":dbl})  [unwired: 1 in]
          }
        }
        n212 = Number To Decimal String(number=w499) -> (decimal integer string=w500:string)  [unwired: 1 in]
        n213 = call "Draw Overlay Point.vi"("Color"=w498, "Cluster"=w497, "Refnum in"=w504) -> ("Refnum out"=w503:T2)  [unwired: 8 in]
        n214 = call "IMAQ Overlay Text"("Text Color (black)"=w498, "String"=w500, "Origin"=w497, "Image"=w503) -> ("Image Out"=w502:T2)  [unwired: 6 in, 1 out]
      }
      n215 = Index Array(array=w457, index #1=1 ("index"), index #2=0 ("index"), index #3=2 ("index")) -> (element #1=w437:cluster{"Position.X":dbl, "Position.Y":dbl}, element #2=w440:cluster{"Position.X":dbl, "Position.Y":dbl}, element #3=w436:cluster{"Position.X":dbl, "Position.Y":dbl})
      n216 = call "IMAQ Overlay Line"("Color"=w439, "End Point"=w437, "Start Point"=w440, "Image"=w446) -> ("Image Out"=w443:T2)  [unwired: 6 in, 1 out]
      n217 = call "IMAQ Overlay Line"("End Point"=w436, "Start Point"=w437, "Image"=w443) -> ("Image Out"=w438:T2)  [unwired: 7 in, 1 out]
      n218 = Unbundle(w437) -> ("Position.X"=w456:dbl, "Position.Y"=w447:dbl)
      n219 = Add(x=w456, y=w455) -> (x+y=w452:dbl)
      n220 = Subtract(x=w447, y=w455) -> (x-y=w453:dbl)
      n221 = Subtract(x=w456, y=w455) -> (x-y=w454:dbl)
      n222 = Add(x=w447, y=w455) -> (x+y=w451:dbl)
      n223 = Bundle(w454, w453, w452, w451) -> (w450:cluster{dbl, dbl, dbl, dbl})  [unwired: 1 in]
      n224 = call "IMAQ Overlay Arc"("End Angle (degrees)"=w445, "Bounding Rectangle"=w450, "Image"=w438) -> ("Image Out"=w458:T2)  [unwired: 7 in, 1 out]
      n225 = disable-structure shown="Enabled" {
        disable-tunnel: [w495 w496] -> w449
        disable-tunnel: "Caliper" -> [w494 _]
        disable-tunnel: w439 -> [w493 _]
        disable-tunnel: w458 -> [w492 w496]
        disable-tunnel: w437 -> [w491 _]
        frame Enabled {
          n226 = call "IMAQ Overlay Text"("Text Color (black)"=w493, "String"=w494, "Origin"=w491, "Image"=w492) -> ("Image Out"=w495:T2)  [unwired: 6 in, 1 out]
        }
        frame Disabled {
        }
      }
      n227 = disable-structure shown="Enabled" {
        disable-tunnel: w449 -> [w489 w490]
        disable-tunnel: [w482 w490] -> w448
        disable-tunnel: w439 -> [w468 _]
        disable-tunnel: w437 -> [w467 _]
        frame Disabled {
          w470 = 10.0 ("x")
          w472 = 10.0 ("x")
          n228 = Unbundle(w467) -> ("Position.X"=w488:dbl, "Position.Y"=w485:dbl)
          n229 = Add(x=50.0, y=w488) -> (x+y=w486:dbl)
          n230 = Bundle(w486, "Position.Y"=w485) -> (w475:cluster{dbl, "Position.Y":dbl})  [unwired: 1 in]
          n231 = call "IMAQ Overlay Line"("Color"=w468, "End Point"=w475, "Start Point"=w467, "Image"=w489) -> ("Image Out"=w484:T2)  [unwired: 6 in, 1 out]
          n232 = Unbundle(w475) -> (w474:dbl, "Position.Y"=w473:dbl)
          n233 = Subtract(x=w474, y=w472) -> (x-y=w481:dbl)
          n234 = Subtract(x=w473, y=w472) -> (x-y=w480:dbl)
          n235 = Bundle(w481, w480) -> (w479:cluster{dbl, dbl})  [unwired: 1 in]
          n236 = call "IMAQ Overlay Line"("Color"=w468, "End Point"=w479, "Start Point"=w475, "Image"=w484) -> ("Image Out"=w483:T2)  [unwired: 6 in, 1 out]
          n237 = Unbundle(w475) -> (w471:dbl, "Position.Y"=w469:dbl)
          n238 = Subtract(x=w471, y=w470) -> (x-y=w477:dbl)
          n239 = Add(x=w469, y=w470) -> (x+y=w478:dbl)
          n240 = Bundle(w477, w478) -> (w476:cluster{dbl, dbl})  [unwired: 1 in]
          n241 = call "IMAQ Overlay Line"("Color"=w468, "End Point"=w476, "Start Point"=w475, "Image"=w483) -> ("Image Out"=w482:T2)  [unwired: 6 in, 1 out]
        }
        frame Enabled {
        }
      }
    }
    frame 7 {
      (unwired) "Caliper"
      n242 = Array Subset(array=w542, length=3) -> (w543:T3[])  [unwired: 1 in]
      n243 = Unbundle By Name(w539) -> ()  [unwired: 1 out]
      n244 = for {
        tunnel: w543 -> [w558] mode=indexing
        tunnel: w541 -> [w556]
        tunnel: w540 -> [w554]
        shift-right: [w550] -> w536
        shift-left: w538 -> [w553]
        tunnel: [w546] -> w527
        tunnel: [w545] -> w537 mode=indexing
        i -> [w549]
        w546 = u32 16711680 ("Text Color (black)")
        n245 = Unbundle By Name(w558) -> ("Type"=w557:T4, "Index"=w555:i32)
        n246 = Increment(x=w549) -> (x+1=w547:i32)
        n247 = case shown="\"AnalysisResult\", Default" w557 {
          tunnel: w556 -> [w566 _]
          tunnel: w555 -> [w565 w574]
          tunnel: [w561 w570] -> w545
          tunnel: w554 -> [_ w569]
          tunnel: [FALSE ("StepError?") w568] -> _
          tunnel: w553 -> [w559 w567]
          tunnel: [w559 w567] -> w552
          frame "AnalysisResult", Default {
            n248 = Index Array(array=w566, index=w565) -> (element=w564:T8)
            n249 = Unbundle By Name(w564) -> ("Position_X"=w563:dbl, "Position_Y"=w562:dbl)
            n250 = Bundle("Position_X"=w563, "Position_Y"=w562) -> (w561:cluster{"Position_X":dbl, "Position_Y":dbl})  [unwired: 1 in]
          }
          frame "CaliperResult" {
            n251 = Index Array(array=w569, index=w574) -> (element=w573:T5)
            n252 = Unbundle By Name(w573) -> ("Result.Position.X"=w572:dbl, "Result.Position.Y"=w571:dbl, "Result.StepError?"=w568:bool)
            n253 = Bundle("Position.X"=w572, "Position.Y"=w571) -> (w570:cluster{"Position.X":dbl, "Position.Y":dbl})  [unwired: 1 in]
          }
        }
        n254 = Number To Decimal String(number=w547) -> (decimal integer string=w548:string)  [unwired: 1 in]
        n255 = call "Draw Overlay Point.vi"("Color"=w546, "Cluster"=w545, "Refnum in"=w552) -> ("Refnum out"=w551:T2)  [unwired: 8 in]
        n256 = call "IMAQ Overlay Text"("Text Color (black)"=w546, "String"=w548, "Origin"=w545, "Image"=w551) -> ("Image Out"=w550:T2)  [unwired: 6 in, 1 out]
      }
      n257 = Index Array(array=w537, index #1=1 ("index"), index #2=0 ("index"), index #3=2 ("index")) -> (element #1=w530:cluster{"Position.X":dbl, "Position.Y":dbl}, element #2=w531:cluster{"Position.X":dbl, "Position.Y":dbl}, element #3=w529:cluster{"Position.X":dbl, "Position.Y":dbl})
      n258 = call "IMAQ Overlay Line"("Color"=w527, "End Point"=w530, "Start Point"=w531, "Image"=w536) -> ("Image Out"=w534:T2)  [unwired: 6 in, 1 out]
      n259 = call "IMAQ Overlay Line"("Color"=w527, "End Point"=w529, "Start Point"=w530, "Image"=w534) -> ("Image Out"=w528:T2)  [unwired: 6 in, 1 out]
    }
    frame 8 {
      w584 = 2.0 ("y")
      n260 = Array Subset(array=w609, length=4) -> (w610:T3[])  [unwired: 1 in]
      n261 = Unbundle By Name(w606) -> ("Position.X"=w599:dbl, "Position.Y"=w598:dbl, "P2.X"=w597:dbl, "P2.Y"=w596:dbl)
      n262 = for {
        tunnel: w610 -> [w625] mode=indexing
        tunnel: w608 -> [w623]
        tunnel: w607 -> [w621]
        shift-right: [w617] -> w603
        shift-left: w605 -> [w620]
        tunnel: [w613] -> w592
        tunnel: [w612] -> w604 mode=indexing
        i -> [w616]
        w613 = u32 16711680 ("Text Color (black)")
        n263 = Unbundle By Name(w625) -> ("Type"=w624:T4, "Index"=w622:i32)
        n264 = Increment(x=w616) -> (x+1=w614:i32)
        n265 = case shown="\"AnalysisResult\", Default" w624 {
          tunnel: w623 -> [w633 _]
          tunnel: w622 -> [w632 w641]
          tunnel: [w628 w637] -> w612
          tunnel: w621 -> [_ w636]
          tunnel: [FALSE ("StepError?") w635] -> _
          tunnel: w620 -> [w626 w634]
          tunnel: [w626 w634] -> w619
          frame "AnalysisResult", Default {
            n266 = Index Array(array=w633, index=w632) -> (element=w631:T8)
            n267 = Unbundle By Name(w631) -> ("Position_X"=w630:dbl, "Position_Y"=w629:dbl)
            n268 = Bundle("Position_X"=w630, "Position_Y"=w629) -> (w628:cluster{"Position_X":dbl, "Position_Y":dbl})  [unwired: 1 in]
          }
          frame "CaliperResult" {
            n269 = Index Array(array=w636, index=w641) -> (element=w640:T5)
            n270 = Unbundle By Name(w640) -> ("Result.Position.X"=w639:dbl, "Result.Position.Y"=w638:dbl, "Result.StepError?"=w635:bool)
            n271 = Bundle("Position.X"=w639, "Position.Y"=w638) -> (w637:cluster{"Position.X":dbl, "Position.Y":dbl})  [unwired: 1 in]
          }
        }
        n272 = Number To Decimal String(number=w614) -> (decimal integer string=w615:string)  [unwired: 1 in]
        n273 = call "Draw Overlay Point.vi"("Color"=w613, "Cluster"=w612, "Refnum in"=w619) -> ("Refnum out"=w618:T2)  [unwired: 8 in]
        n274 = call "IMAQ Overlay Text"("Text Color (black)"=w613, "String"=w615, "Origin"=w612, "Image"=w618) -> ("Image Out"=w617:T2)  [unwired: 6 in, 1 out]
      }
      n275 = Bundle("P2.X"=w597, "P2.Y"=w596) -> (w580:cluster{"P2.X":dbl, "P2.Y":dbl})  [unwired: 1 in]
      n276 = Bundle("Position.X"=w599, "Position.Y"=w598) -> (w581:cluster{"Position.X":dbl, "Position.Y":dbl})  [unwired: 1 in]
      n277 = Index Array(array=w604) -> (element #1=w578:cluster{"Position.X":dbl, "Position.Y":dbl}, element #2=w577:cluster{"Position.X":dbl, "Position.Y":dbl}, element #3=w576:cluster{"Position.X":dbl, "Position.Y":dbl}, element #4=w575:cluster{"Position.X":dbl, "Position.Y":dbl})  [unwired: 4 in]
      n278 = call "IMAQ Overlay Line"("Color"=w592, "End Point"=w577, "Start Point"=w578, "Image"=w603) -> ("Image Out"=w602:T2)  [unwired: 6 in, 1 out]
      n279 = call "IMAQ Overlay Line"("Color"=w592, "End Point"=w575, "Start Point"=w576, "Image"=w602) -> ("Image Out"=w601:T2)  [unwired: 6 in, 1 out]
      n280 = call "Draw Overlay Point.vi"("Color"=w592, "Cluster"=w581, "Refnum in"=w601) -> ("Refnum out"=w600:T2)  [unwired: 8 in]
      n281 = call "Draw Overlay Point.vi"("Color"=w592, "Cluster"=w580, "Refnum in"=w600) -> ("Refnum out"=w595:T2)  [unwired: 8 in]
      n282 = Unbundle(w581) -> ("Position.X"=w590:dbl, "Position.Y"=w587:dbl)
      n283 = Unbundle(w580) -> ("P2.X"=w588:dbl, "P2.Y"=w589:dbl)
      n284 = Add(x=w590, y=w588) -> (x+y=w586:dbl)
      n285 = Add(x=w587, y=w589) -> (x+y=w585:dbl)
      n286 = call "IMAQ Overlay Line"("Color"=w592, "End Point"=w580, "Start Point"=w581, "Image"=w595) -> ("Image Out"=w594:T2)  [unwired: 6 in, 1 out]
      n287 = Divide(x=w586, y=w584) -> (x/y=w583:dbl)
      n288 = Divide(x=w585, y=w584) -> (x/y=w582:dbl)
      n289 = Bundle(w583, w582) -> (w579:cluster{dbl, dbl})  [unwired: 1 in]
      n290 = call "IMAQ Overlay Text"("Text Color (black)"=w592, "String"="Caliper", "Origin"=w579, "Image"=w594) -> ("Image Out"=w593:T2)  [unwired: 6 in, 1 out]
    }
    frame 11 {
      w651 = 2.0 ("y")
      n291 = Array Subset(array=w676, length=4) -> (w677:T3[])  [unwired: 1 in]
      n292 = Unbundle By Name(w673) -> ("Position.X"=w666:dbl, "Position.Y"=w665:dbl, "P2.X"=w664:dbl, "P2.Y"=w663:dbl)
      n293 = for {
        tunnel: w677 -> [w692] mode=indexing
        tunnel: w675 -> [w690]
        tunnel: w674 -> [w688]
        shift-right: [w684] -> w670
        shift-left: w672 -> [w687]
        tunnel: [w680] -> w659
        tunnel: [w679] -> w671 mode=indexing
        i -> [w683]
        w680 = u32 16711680 ("Text Color (black)")
        n294 = Unbundle By Name(w692) -> ("Type"=w691:T4, "Index"=w689:i32)
        n295 = Increment(x=w683) -> (x+1=w681:i32)
        n296 = case shown="\"AnalysisResult\", Default" w691 {
          tunnel: w690 -> [w700 _]
          tunnel: w689 -> [w699 w708]
          tunnel: [w695 w704] -> w679
          tunnel: w688 -> [_ w703]
          tunnel: [FALSE ("StepError?") w702] -> _
          tunnel: w687 -> [w693 w701]
          tunnel: [w693 w701] -> w686
          frame "AnalysisResult", Default {
            n297 = Index Array(array=w700, index=w699) -> (element=w698:T8)
            n298 = Unbundle By Name(w698) -> ("Position_X"=w697:dbl, "Position_Y"=w696:dbl)
            n299 = Bundle("Position_X"=w697, "Position_Y"=w696) -> (w695:cluster{"Position_X":dbl, "Position_Y":dbl})  [unwired: 1 in]
          }
          frame "CaliperResult" {
            n300 = Index Array(array=w703, index=w708) -> (element=w707:T5)
            n301 = Unbundle By Name(w707) -> ("Result.Position.X"=w706:dbl, "Result.Position.Y"=w705:dbl, "Result.StepError?"=w702:bool)
            n302 = Bundle("Position.X"=w706, "Position.Y"=w705) -> (w704:cluster{"Position.X":dbl, "Position.Y":dbl})  [unwired: 1 in]
          }
        }
        n303 = Number To Decimal String(number=w681) -> (decimal integer string=w682:string)  [unwired: 1 in]
        n304 = call "Draw Overlay Point.vi"("Color"=w680, "Cluster"=w679, "Refnum in"=w686) -> ("Refnum out"=w685:T2)  [unwired: 8 in]
        n305 = call "IMAQ Overlay Text"("Text Color (black)"=w680, "String"=w682, "Origin"=w679, "Image"=w685) -> ("Image Out"=w684:T2)  [unwired: 6 in, 1 out]
      }
      n306 = Bundle("P2.X"=w664, "P2.Y"=w663) -> (w647:cluster{"P2.X":dbl, "P2.Y":dbl})  [unwired: 1 in]
      n307 = Bundle("Position.X"=w666, "Position.Y"=w665) -> (w648:cluster{"Position.X":dbl, "Position.Y":dbl})  [unwired: 1 in]
      n308 = Index Array(array=w671) -> (element #1=w645:cluster{"Position.X":dbl, "Position.Y":dbl}, element #2=w644:cluster{"Position.X":dbl, "Position.Y":dbl}, element #3=w643:cluster{"Position.X":dbl, "Position.Y":dbl}, element #4=w642:cluster{"Position.X":dbl, "Position.Y":dbl})  [unwired: 4 in]
      n309 = call "IMAQ Overlay Line"("Color"=w659, "End Point"=w644, "Start Point"=w645, "Image"=w670) -> ("Image Out"=w669:T2)  [unwired: 6 in, 1 out]
      n310 = call "IMAQ Overlay Line"("Color"=w659, "End Point"=w642, "Start Point"=w643, "Image"=w669) -> ("Image Out"=w668:T2)  [unwired: 6 in, 1 out]
      n311 = call "Draw Overlay Point.vi"("Color"=w659, "Cluster"=w648, "Refnum in"=w668) -> ("Refnum out"=w667:T2)  [unwired: 8 in]
      n312 = call "Draw Overlay Point.vi"("Color"=w659, "Cluster"=w647, "Refnum in"=w667) -> ("Refnum out"=w662:T2)  [unwired: 8 in]
      n313 = Unbundle(w648) -> ("Position.X"=w657:dbl, "Position.Y"=w654:dbl)
      n314 = Unbundle(w647) -> ("P2.X"=w655:dbl, "P2.Y"=w656:dbl)
      n315 = Add(x=w657, y=w655) -> (x+y=w653:dbl)
      n316 = Add(x=w654, y=w656) -> (x+y=w652:dbl)
      n317 = call "IMAQ Overlay Line"("Color"=w659, "End Point"=w647, "Start Point"=w648, "Image"=w662) -> ("Image Out"=w661:T2)  [unwired: 6 in, 1 out]
      n318 = Divide(x=w653, y=w651) -> (x/y=w650:dbl)
      n319 = Divide(x=w652, y=w651) -> (x/y=w649:dbl)
      n320 = Bundle(w650, w649) -> (w646:cluster{dbl, dbl})  [unwired: 1 in]
      n321 = call "IMAQ Overlay Text"("Text Color (black)"=w659, "String"="Caliper", "Origin"=w646, "Image"=w661) -> ("Image Out"=w660:T2)  [unwired: 6 in, 1 out]
    }
    frame 9 {
      w717 = 2.0 ("y")
      # "輸出中線"
      # "Mid Line"
      n322 = Array Subset(array=w740, length=4) -> (w741:T3[])  [unwired: 1 in]
      n323 = Unbundle By Name(w737) -> ("Position.X"=w732:dbl, "Position.Y"=w731:dbl, "P2.X"=w730:dbl, "P2.Y"=w729:dbl)
      n324 = for {
        tunnel: w741 -> [w756] mode=indexing
        tunnel: w739 -> [w754]
        tunnel: w738 -> [w752]
        shift-right: [w748] -> w734
        shift-left: w736 -> [w751]
        tunnel: [w744] -> w725
        tunnel: [w743] -> w735 mode=indexing
        i -> [w747]
        w744 = u32 16711680 ("Text Color (black)")
        n325 = Unbundle By Name(w756) -> ("Type"=w755:T4, "Index"=w753:i32)
        n326 = Increment(x=w747) -> (x+1=w745:i32)
        n327 = case shown="\"AnalysisResult\", Default" w755 {
          tunnel: w754 -> [w764 _]
          tunnel: w753 -> [w763 w772]
          tunnel: [w759 w768] -> w743
          tunnel: w752 -> [_ w767]
          tunnel: [FALSE ("StepError?") w766] -> _
          tunnel: w751 -> [w757 w765]
          tunnel: [w757 w765] -> w750
          frame "AnalysisResult", Default {
            n328 = Index Array(array=w764, index=w763) -> (element=w762:T8)
            n329 = Unbundle By Name(w762) -> ("Position_X"=w761:dbl, "Position_Y"=w760:dbl)
            n330 = Bundle("Position_X"=w761, "Position_Y"=w760) -> (w759:cluster{"Position_X":dbl, "Position_Y":dbl})  [unwired: 1 in]
          }
          frame "CaliperResult" {
            n331 = Index Array(array=w767, index=w772) -> (element=w771:T5)
            n332 = Unbundle By Name(w771) -> ("Result.Position.X"=w770:dbl, "Result.Position.Y"=w769:dbl, "Result.StepError?"=w766:bool)
            n333 = Bundle("Position.X"=w770, "Position.Y"=w769) -> (w768:cluster{"Position.X":dbl, "Position.Y":dbl})  [unwired: 1 in]
          }
        }
        n334 = Number To Decimal String(number=w745) -> (decimal integer string=w746:string)  [unwired: 1 in]
        n335 = call "Draw Overlay Point.vi"("Color"=w744, "Cluster"=w743, "Refnum in"=w750) -> ("Refnum out"=w749:T2)  [unwired: 8 in]
        n336 = call "IMAQ Overlay Text"("Text Color (black)"=w744, "String"=w746, "Origin"=w743, "Image"=w749) -> ("Image Out"=w748:T2)  [unwired: 6 in, 1 out]
      }
      n337 = Bundle("P2.X"=w730, "P2.Y"=w729) -> (w713:cluster{"P2.X":dbl, "P2.Y":dbl})  [unwired: 1 in]
      n338 = Bundle("Position.X"=w732, "Position.Y"=w731) -> (w714:cluster{"Position.X":dbl, "Position.Y":dbl})  [unwired: 1 in]
      n339 = Index Array(array=w735) -> (element #1=w711:cluster{"Position.X":dbl, "Position.Y":dbl}, element #2=w710:cluster{"Position.X":dbl, "Position.Y":dbl})  [unwired: 2 in]
      n340 = call "IMAQ Overlay Line"("Color"=w725, "End Point"=w710, "Start Point"=w711, "Image"=w734) -> ("Image Out"=w709:T2)  [unwired: 6 in, 1 out]
      n341 = call "Draw Overlay Point.vi"("Color"=w725, "Cluster"=w714, "Refnum in"=w709) -> ("Refnum out"=w733:T2)  [unwired: 8 in]
      n342 = call "Draw Overlay Point.vi"("Color"=w725, "Cluster"=w713, "Refnum in"=w733) -> ("Refnum out"=w728:T2)  [unwired: 8 in]
      n343 = Unbundle(w714) -> ("Position.X"=w723:dbl, "Position.Y"=w720:dbl)
      n344 = Unbundle(w713) -> ("P2.X"=w721:dbl, "P2.Y"=w722:dbl)
      n345 = Add(x=w723, y=w721) -> (x+y=w719:dbl)
      n346 = Add(x=w720, y=w722) -> (x+y=w718:dbl)
      n347 = call "IMAQ Overlay Line"("Color"=w725, "End Point"=w713, "Start Point"=w714, "Image"=w728) -> ("Image Out"=w727:T2)  [unwired: 6 in, 1 out]
      n348 = Divide(x=w719, y=w717) -> (x/y=w716:dbl)
      n349 = Divide(x=w718, y=w717) -> (x/y=w715:dbl)
      n350 = Bundle(w716, w715) -> (w712:cluster{dbl, dbl})  [unwired: 1 in]
      n351 = call "IMAQ Overlay Text"("Text Color (black)"=w725, "String"="Caliper", "Origin"=w712, "Image"=w727) -> ("Image Out"=w726:T2)  [unwired: 6 in, 1 out]
    }
  }
  "Image Out" <- w3
